vi "Pack for gRPC.vi"(8 "error in":errorcluster, 9 "configuration / results":enum16{"Configuration", "Results"}(ring), 10 "data value":variant, 11 "measurement plugin in":refnum<class "FPT_SParam.lvclass">) -> (0 "error out":errorcluster, 2 "any":T1, 3 "measurement plugin out":refnum<class "FPT_SParam.lvclass">)   [LabVIEW 2023, in "FPT_SParam.lvclass"]
uses:
  FPT_SParam.lvclass
  <vilib>/gRPC/LabVIEW gRPC Library/Shared/Any.ctl
  C:/Program Files/National Instruments/LabVIEW 2023/vi.lib/Plug-In SDKs/Measurements/Measurement Plugin Service/Measurement Plugin Service.lvclass
  Measurement Configuration.ctl
  Measurement Results.ctl
  2eca732d-dbaa-43bf-a7dd-ede2da65bc1b.vi
  a6012965-5700-4384-8228-972e71b6560c.vi
  <vilib>/gRPC/LabVIEW gRPC Library/Server API/Translate Protobuf Error.vi
  <vilib>/AdvancedString/1D String Array to Delimited String.vi
  <vilib>/gRPC/LabVIEW gRPC Library/Server API/Server/Get Server DLL Path.vi
  FPT_SParam.lvclass/FPT_SParam.ctl
  <vilib>/Plug-In SDKs/Measurements/Measurement Plugin Service/Measurement Plugin Service.lvclass
  <vilib>/gRPC/LabVIEW gRPC Library/grpc-lvsupport-release.lvlib
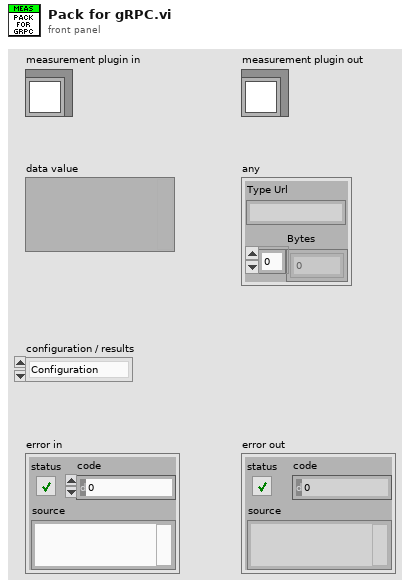
[diagram p1: front panel]
types:
  T1 = typedef "grpc-lvsupport-release.lvlib/Any.ctl" = cluster{"Type Url":string, "Bytes":u8[]}
  T2 = typedef "grpc-lvsupport-release.lvlib/grpcId.ctl" = u64
  T3 = typedef "FPT_SParam.lvclass/Measurement Configuration.ctl" = cluster{"Automation Test":bool, "Power sequencing file path":string, "RFmxVNA name":string, "vCal Name":string, "RFmxVNA Calset Enable":bool, "RFmxVNA Calset Interpolation":bool, "Calset File Path (String)":string, "RFmxVNA attenuation mode":enum32{"<None>", "s2p File"}, "RFmxVNA Port1 s2p file path (String)":string, "RFmxVNA Port1 s-parameters orientation":enum32{"Port1 Towards DUT", "Port2 Towards DUT"}, "RFmxVNA Port1 Power Compensation":bool, "RFmxVNA Port2 s2p file path (String)":string, "RFmxVNA Port2 s-parameters orientation":enum32{"Port1 Towards DUT", "Port2 Towards DUT"}, "RFmxVNA Port2 Power Compensation":bool, "Port1 Power Level (dBm)":dbl, "Port1 Test Receiver Attenuation (dB)":dbl, "Port2 Power Level (dBm)":dbl, "Port2 Test Receiver Attenuation (dB)":dbl, "IF Bandwidth (Hz)":dbl, "Action":enum32{"Calibrate", "Measure"}, "Pulse Mode Enabled":bool, "Pulse Period":dbl, "Pulse Modulator Delay":dbl, "Pulse Modulator Width":dbl, "Pulse Acquisition Auto":bool, "Pulse Acquisition Delay":dbl, "Pulse Acquisition Width":dbl, "Start Frequency (Hz)":dbl, "Stop Frequency (Hz)":dbl, "Number of Points":i32, "Measurement S-Parameters":string[], "Phase Trace Type":i32, "Magnitude Units":i32, "SnP File Path (String)":string, "Averaging Enabled":bool, "Averaging Count":u32}
  T4 = typedef "FPT_SParam.lvclass/Measurement Results.ctl" = cluster{"Status":string, "S-Param Name":string[], "S-Param Magnitude":dbl[][], "S-Param Phase":dbl[][], "VNA Status":string}
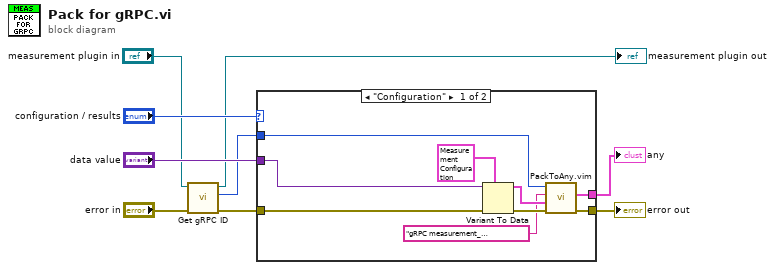
[diagram p0: block diagram]
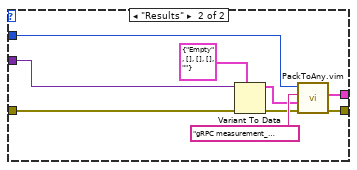
[diagram p2: hidden frame]
diagram:
  n1 = call <vilib>:"Get gRPC ID.vi"("error in"="error in", "measurement plugin service in"="measurement plugin in") -> ("error out"=w4:errorcluster, "gRPC ID"=w1:T2, "measurement plugin service out"=→"measurement plugin out":refnum<class "FPT_SParam.lvclass">)  [unwired: 7 in]
  n2 = case shown="\"Configuration\"" "configuration / results" {
    tunnel: w4 -> [w18 w27]
    tunnel: "data value" -> [w17 w26]
    tunnel: w1 -> [w14 w22]
    tunnel: [w16 w24] -> w8
    tunnel: [w15 w23] -> w7
    frame "Configuration" {
      n3 = Variant To Data(error in=w18, type=T3 {"Automation Test"=FALSE, "Power sequencing file path"="Lorem ipsum dolor sit", "RFmxVNA name"="5842_0", "vCal Name"="", "RFmxVNA Calset Enable"=FALSE, "RFmxVNA Calset Interpolation"=FALSE, "Calset File Path (String)"="", "RFmxVNA attenuation mode"=enum."s2p File", "RFmxVNA Port1 s2p file path (String)"="", "RFmxVNA Port1 s-parameters orientation"=enum."Port1 Towards DUT", "RFmxVNA Port1 Power Compensation"=FALSE, "RFmxVNA Port2 s2p file path (String)"="", "RFmxVNA Port2 s-parameters orientation"=enum."Port1 Towards DUT", "RFmxVNA Port2 Power Compensation"=FALSE, "Port1 Power Level (dBm)"=1.0, "Port1 Test Receiver Attenuation (dB)"=1.0, "Port2 Power Level (dBm)"=1.0, "Port2 Test Receiver Attenuation (dB)"=1.0, "IF Bandwidth (Hz)"=1.0, "Action"=enum."Measure", "Pulse Mode Enabled"=FALSE, "Pulse Period"=0.001, "Pulse Modulator Delay"=0.0, "Pulse Modulator Width"=0.0001, "Pulse Acquisition Auto"=FALSE, "Pulse Acquisition Delay"=2e-05, "Pulse Acquisition Width"=4.665e-05, "Start Frequency (Hz)"=4000000000.0, "Stop Frequency (Hz)"=26000000000.0, "Number of Points"=200, "Measurement S-Parameters"=["S11", "S12", "S21", "S22"], "Phase Trace Type"=0, "Magnitude Units"=0, "SnP File Path (String)"="", "Averaging Enabled"=FALSE, "Averaging Count"=0} ("measurement configuration"), Variant=w17) -> (data=w13:T3, error out=w12:errorcluster)
      n4 = call "PackToAny.vim"("error in"=w12, "Data To Pack"=w13, "Message Type"="gRPC measurement_measurement configuration", "gRPCid in"=w14) -> ("error out"=w16:errorcluster, "Any"=w15:T1)  [unwired: 5 in, 1 out]
    }
    frame "Results" {
      n5 = Variant To Data(error in=w27, type=T4 {"Status"="Empty", "S-Param Name"=[], "S-Param Magnitude"=[], "S-Param Phase"=[], "VNA Status"=""} ("Measurement Results"), Variant=w26) -> (data=w20:T4, error out=w19:errorcluster)
      n6 = call "PackToAny.vim"("error in"=w19, "Data To Pack"=w20, "Message Type"="gRPC measurement_measurement results", "gRPCid in"=w22) -> ("error out"=w24:errorcluster, "Any"=w23:T1)  [unwired: 5 in, 1 out]
    }
  }
  "error out" <- w8
  "any" <- w7
